vi "sub vi - Step Piezo Read Strain Gauge.vi"() -> ()   [LabVIEW 2010]
uses:
  <vilib>/DAQmx/read.llb/DAQmx Read (Analog DBL 1Chan 1Samp).vi
  <vilib>/DAQmx/create/channels.llb/DAQmx Create Channel (AI-Voltage-Basic).vi
  <vilib>/daqmx/miscellaneous.llb/DAQmx Fill In Error Info.vi
  <vilib>/Utility/file.llb/Write To Spreadsheet File (DBL).vi
panel:
  out "Waveform Chart":dbl(graph)
  out "Waveform Graph":dbl[](graph)
  in  "Save Data":bool
  in  "Data File Name":path=path "StepResolution.txt" caption="File Name"
  in  "# of Steps":i32=20
  in  "# measurements":i32=100
  in  "Measure Wait":u32=10
  in  "Step Size":dbl=0.001
  in  "Start":dbl
  in  "Axis":u16(ring)=2 items=["X", "Y", "Z"]
  out "X Position":dbl
  out "Y Position":dbl
  out "Z Position":dbl
  in  "Move Wait":u32=10
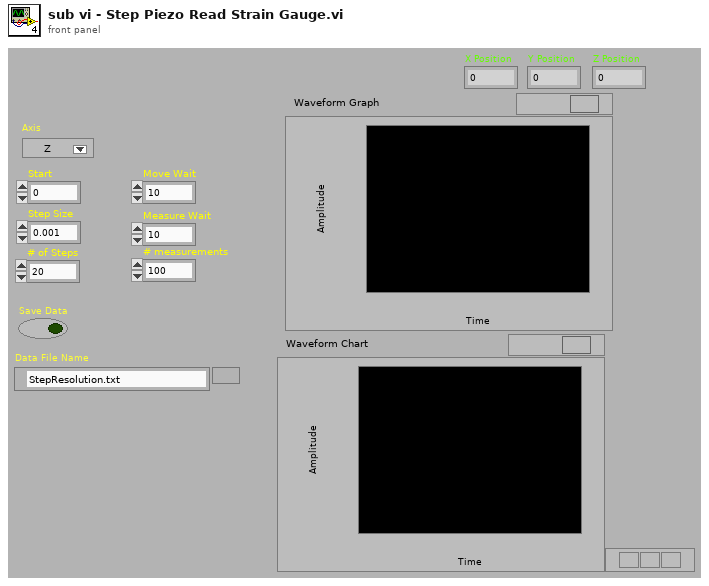
[diagram p1: front panel]
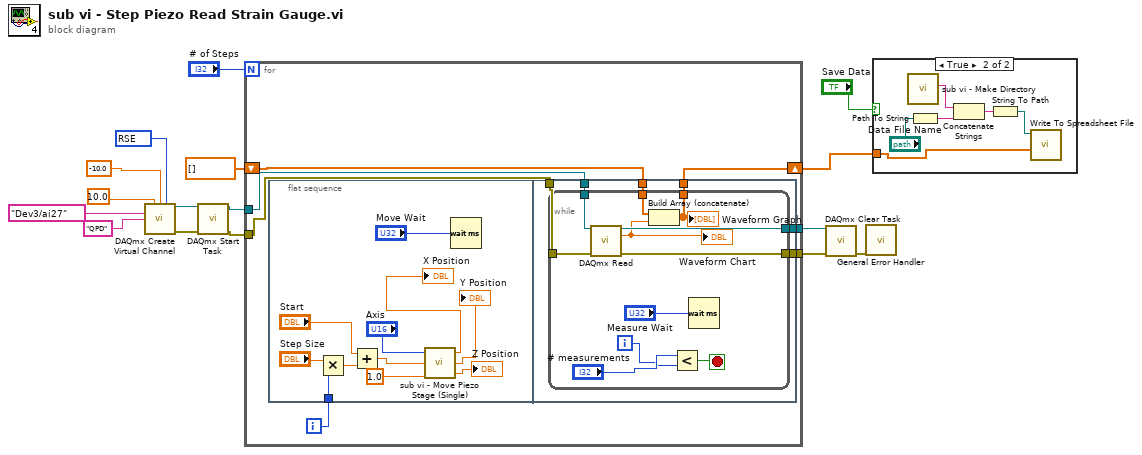
[diagram p0: block diagram]
diagram:
  w14 = 10083 items=["default"=-1, "RSE"=10083, "NRSE"=10078, "Differential"=10106, "Pseudodifferential"=12529] ("input terminal configuration")
  n1 = call-poly <vilib>:"DAQmx Create Virtual Channel.vi"("maximum value"=10.0, "minimum value"=-10.0, "input terminal configuration"=w14, "physical channels"=tag "Dev3/ai27", "name to assign"="QPD") -> ("task out"=w13:refnum<k21>, "error out"=w12:errorcluster)  [unwired: 4 in, 5 out]
  n2 = call <vilib>:"DAQmx Start Task.vi"("task/channels in"=w13, "error in"=w12) -> ("task out"=w10:refnum<k21>, "error out"=w9:errorcluster)  [unwired: 12 out]
  n3 = for {
    N: "# of Steps" -> [_]
    tunnel: w10 -> [w20]
    tunnel: w9 -> [w19]
    tunnel: [w22] -> w5
    tunnel: [w21] -> w4
    shift-right: [w18] -> w1
    shift-left: dbl[] [] -> [w17]
    i -> [w23]
    n4 = flat-sequence {
      tunnel: w23 -> [w34]
      tunnel: [w40] -> w22
      tunnel: [w39] -> w21
      tunnel: w20 -> [w38]
      tunnel: [w37] -> _
      tunnel: w19 -> [w37]
      tunnel: [w36] -> w18
      tunnel: w17 -> [w35]
      frame #0 {
        n5 = Multiply(x="Step Size", y=w34) -> (x*y=w32:dbl)
        n6 = Add(x="Start", y=w32) -> (x+y=w28:dbl)
        n7 = call "sub vi - Move Piezo Stage (Single).vi"("frequency"=1.0, "Desired Position (um)"=w28, "Axis"="Axis") -> ("Z Position"=→"Z Position":dbl, "Y Position"=→"Y Position":dbl, "X Position"=→"X Position":dbl)
        n8 = Wait (ms)(milliseconds to wait="Move Wait") -> ()  [unwired: 1 out]
      }
      frame #1 {
        n9 = while {
          tunnel: [w51] -> w40
          tunnel: [w50] -> w39
          tunnel: w38 -> [w49]
          tunnel: w37 -> [w48]
          tunnel: [w43] -> w36
          tunnel: w35 -> [w42]
          i -> [w45]
          stop <- w47 stop-if-true
          n10 = call-poly <vilib>:"DAQmx Read.vi"("task/channels in"=w49, "error in"=w48) -> ("task out"=w51:refnum<k21>, "data"=w41:dbl, "error out"=w50:errorcluster)  [unwired: 1 in, 10 out]
          "Waveform Chart" <- w41
          n11 = Build Array (concatenate)(w42, w41) -> (w43:dbl[])
          "Waveform Graph" <- w43
          n12 = Less?(x="# measurements", y=w45) -> (x < y?=w47:bool)
          n13 = Wait (ms)(milliseconds to wait="Measure Wait") -> ()  [unwired: 1 out]
        }
      }
    }
  }
  n14 = call <vilib>:"DAQmx Clear Task.vi"("task in"=w5, "error in"=w4) -> ("error out"=w11:errorcluster)  [unwired: 13 out]
  n15 = call <vilib>:"General Error Handler.vi"("error in (no error)"=w11) -> ()  [unwired: 2 in, 13 out]
  n16 = case shown="True" "Save Data" {
    tunnel: w1 -> [_ w52]
    frame False {
    }
    frame True {
      n17 = call "sub vi - Make Directory.vi"() -> ("directory"=w53:string)  [unwired: 2 in, 9 out]
      n18 = Path To String(path="Data File Name") -> (string=w56:string)
      n19 = Concatenate Strings(w53, w56) -> (w57:string)
      n20 = String To Path(string=w57) -> (path=w55:path)
      n21 = call-poly <vilib>:"Write To Spreadsheet File.vi"("1D data"=w52, "file path (dialog if empty)"=w55) -> ()  [unwired: 4 in, 3 out]
    }
  }
